vi "SetDataFolder.vi"(0 "User Data Folder":path, 2 "JustKillAllSavedReferences(False)":bool, 5 "error in (no error)":errorcluster, 6 "WebView2Control ID":i32, 8 "Webview container":refnum<k24>) -> (14 "Environment":refnum<k24>, 15 "UserDataFolder":string="C:\\ProgramData\\LcWebVIEW", 16 "Error Message":string, 19 "error out":errorcluster)   [LabVIEW 2020, in "DP_WebView.lvclass"]
uses:
  DP_WebView.lvclass
  C:/Projects/DependencyViewer/DependencyViewer/DP_WebView_class/data/Microsoft.Web.WebView2.Core.dll
  data/Microsoft.Web.WebView2.Core.dll
  C:/Projects/DependencyViewer/DependencyViewer/DP_WebView_class/data/Microsoft.Web.WebView2.WinForms.dll
  data/Microsoft.Web.WebView2.WinForms.dll
  <vilib>/Utility/sysdir.llb/System Directory Type.ctl
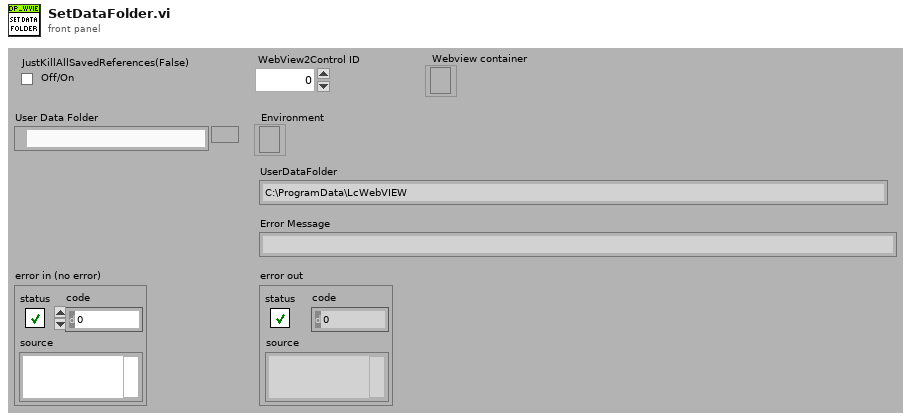
[diagram p1: front panel]
types:
  T1 = typedef "System Directory Type.ctl" = i32
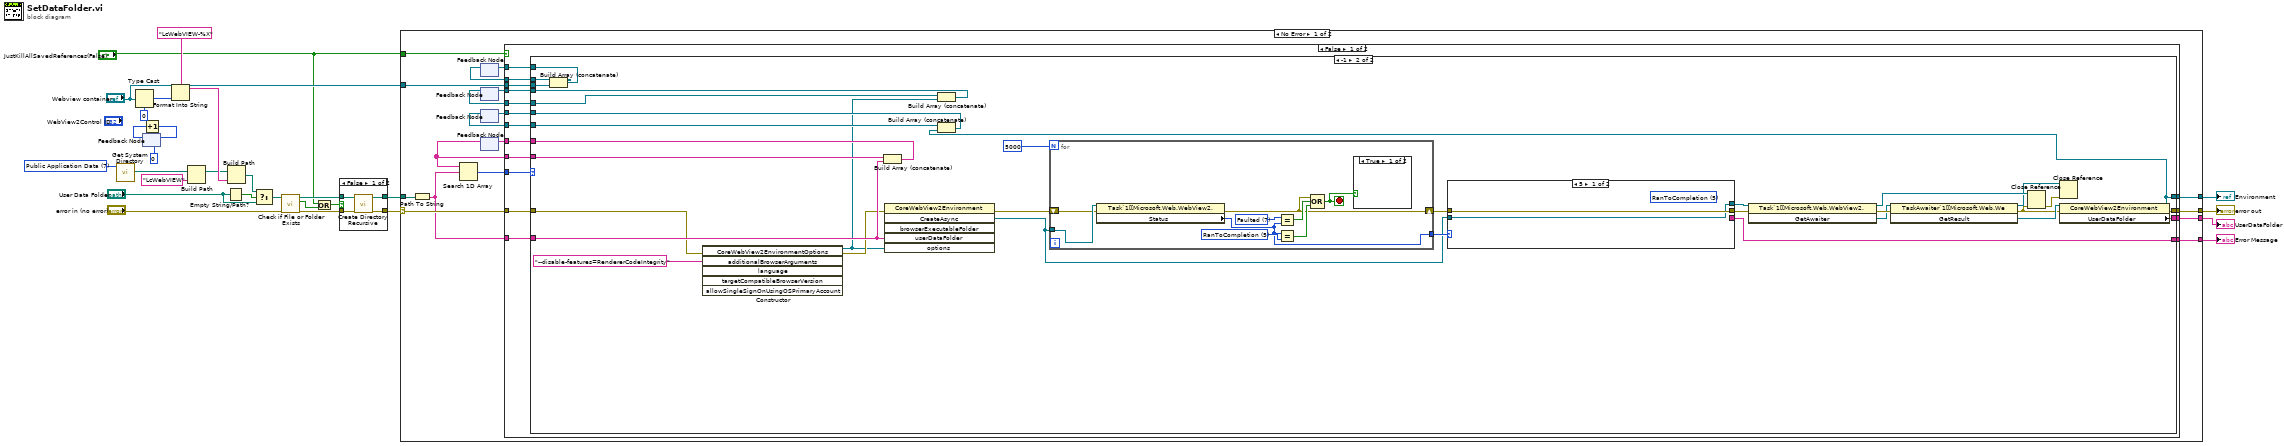
[diagram p0: block diagram]
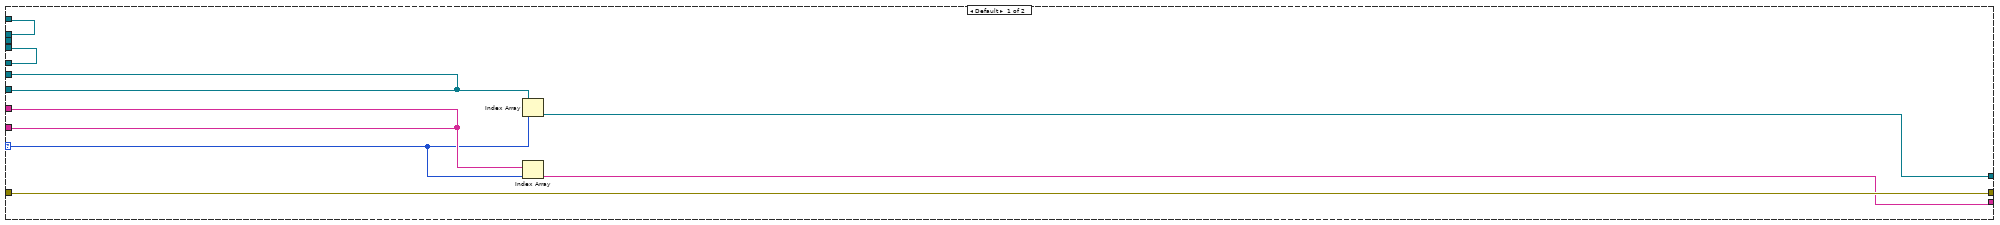
[diagram p3: hidden frame]
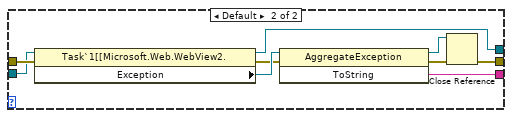
[diagram p4: hidden frame]
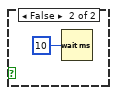
[diagram p5: hidden frame]
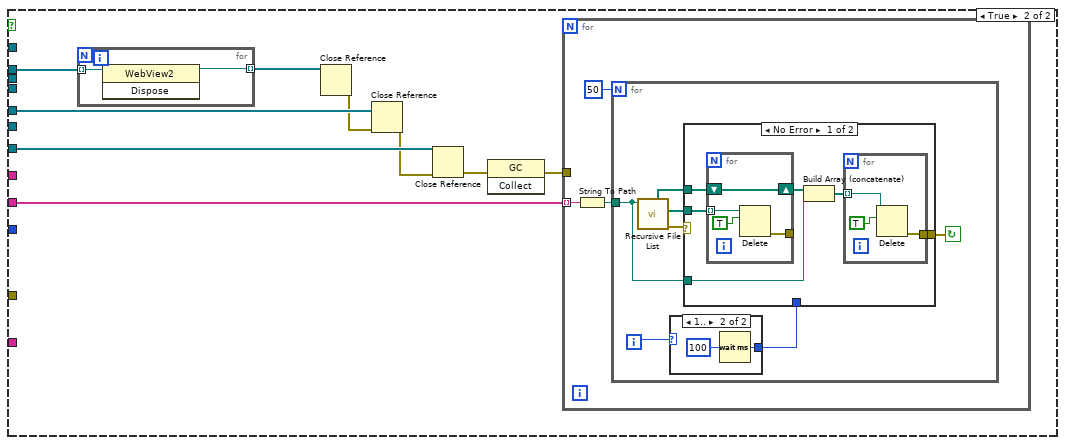
[diagram p6: hidden frame]
diagram:
  w25 = T1 7 items=["User Home"=0, "User Desktop"=1, "User Documents"=2, "User Application Data"=3, "User Preferences"=4, "User Temporary"=5, "Public Documents"=6, "Public Application Data"=7, "Public Preferences"=8, "Public Cache"=13, "System Core Libraries"=9, "System Installed Libraries"=10, "Application Files"=11, "Boot Volume Root"=12] ("system directory type")
  n1 = call <vilib>:"Get System Directory.vi"("system directory type"=w25) -> ("system directory"=w11:path)  [unwired: 10 in]
  n2 = Type Cast(type=u32 0 ("WebView2Control ID"), x="Webview container") -> (*(type *) &x=w4:u32)
  n3 = feedback #1(u32 0 ("WebView2Control ID")) -> (w7:u32)
  n4 = Increment(x=w7) -> (x+1=w6:u32)
  n5 = feedback-in #1(w6) -> ()
  n6 = Format Into String(format string="LcWebVIEW-%X", w4) -> (resulting string=w12:string)  [unwired: 2 in, 1 out]
  n7 = Build Path(base path=w11, name or relative path="LcWebVIEW") -> (appended path=w10:path)
  n8 = Empty String/Path?(string/path="User Data Folder") -> (empty?=w17:bool)
  n9 = Build Path(base path=w10, name or relative path=w12) -> (appended path=w15:path)
  n10 = Select(t=w15, s=w17, f="User Data Folder") -> (s? t:f=w14:path)
  n11 = call <vilib>:"Check if File or Folder Exists.vi"("error in (no error)"="error in (no error)", "path"=w14) -> ("error out"=w28:errorcluster, "file or folder exists?"=w26:bool, "dup path"=w27:path)  [unwired: 7 in]
  n12 = Or(x="JustKillAllSavedReferences(False)", y=w26) -> (x .or. y?=w2:bool)
  n13 = case shown="False" w2 {
    tunnel: w27 -> [w32 w33]
    tunnel: w28 -> [w31 w34]
    tunnel: [w30 w34] -> w23
    tunnel: [w29 w33] -> w22
    frame False {
      n14 = call <vilib>:"Create Directory Recursive.vi"("error in (no error)"=w31, "directory"=w32) -> ("error out"=w30:errorcluster, "directory copy"=w29:path)  [unwired: 3 in, 1 out]
    }
    frame True {
    }
  }
  n15 = case shown="No Error" w23 {
    selector: w23 -> [w52 w166]
    tunnel: w22 -> [w51 _]
    tunnel: [w49 w166] -> w21
    tunnel: [w50 _] -> w20
    tunnel: [w47 _] -> w19
    tunnel: [w48 _] -> w18
    tunnel: "JustKillAllSavedReferences(False)" -> [w38 _]
    tunnel: "Webview container" -> [w35 _]
    frame No Error {
      n16 = Path To String(path=w51) -> (string=w46:string)
      n17 = feedback #2() -> (w36:refnum<k24>[])  [unwired: 1 in]
      n18 = feedback #3() -> (w39:refnum<k24>[])  [unwired: 1 in]
      n19 = feedback #4() -> (w42:refnum<k24>[])  [unwired: 1 in]
      n20 = feedback #5() -> (w44:string[])  [unwired: 1 in]
      n21 = Search 1D Array(1D array=w44, element=w46) -> (index of element=w45:i32)  [unwired: 1 in]
      n22 = case shown="False" w38 {
        tunnel: w52 -> [w68 _]
        tunnel: [w67 _] -> w50
        tunnel: [w66 _] -> w49
        tunnel: [w65 _] -> w48
        tunnel: [w64 _] -> w47
        tunnel: w46 -> [w63 _]
        tunnel: w45 -> [w62 _]
        tunnel: w44 -> [w61 w133]
        tunnel: [w60 _] -> w43
        tunnel: w42 -> [w59 w138]
        tunnel: [w58 _] -> w41
        tunnel: [w57 _] -> w40
        tunnel: w39 -> [w56 w137]
        tunnel: [w54 _] -> w37
        tunnel: w36 -> [w55 w136]
        tunnel: w35 -> [w53 _]
        frame False {
          n23 = case shown="-1" w62 {
            selector: w62 -> [w72 _]
            tunnel: w68 -> [w74 w77]
            tunnel: [w71 w108] -> w67
            tunnel: [w74 w101] -> w66
            tunnel: [w75 w86] -> w65
            tunnel: [_ w99] -> w64
            tunnel: w63 -> [_ w92]
            tunnel: w61 -> [w73 w93]
            tunnel: [w73 w91] -> w60
            tunnel: w59 -> [w76 w90]
            tunnel: [w76 w89] -> w58
            tunnel: w56 -> [w70 w85]
            tunnel: [w70 w81] -> w57
            tunnel: w55 -> [w69 w84]
            tunnel: [w69 w82] -> w54
            tunnel: w53 -> [_ w83]
            frame Default {
              n24 = Index Array(array=w76, index=w72) -> (element=w75:refnum<k24>)
              n25 = Index Array(array=w73, index=w72) -> (element=w71:string)
            }
            frame -1 {
              n26 = Build Array (concatenate)(w84, w83) -> (w82:refnum<k24>[])
              n27 = constructor class="CoreWebView2EnvironmentOptions"(error in=w77, "additionalBrowserArguments"="--disable-features=RendererCodeIntegrity" ("AdditionalBrowserArguments")) -> (reference out=w79:refnum<k24>, error out=w87:errorcluster)  [unwired: 5 in, 5 out]
              n28 = Build Array (concatenate)(w93, w92) -> (w91:string[])
              n29 = invoke class="CoreWebView2Environment" method="CreateAsync"(error in=w87, "userDataFolder"=w92, "options"=w79) -> (error out=w78:errorcluster, "CreateAsync"=w80:refnum<k24>)  [unwired: 3 in, 4 out]
              n30 = Build Array (concatenate)(w85, w79) -> (w81:refnum<k24>[])
              n31 = for {
                N: 5000 -> [_]
                tunnel: w80 -> [w128]
                shift-right: [w122] -> w100
                shift-left: w78 -> [w127]
                tunnel: [w121] -> w96
                stop <- w120 stop-if-true
                w125 = 5 items=["Created", "WaitingForActivation", "WaitingToRun", "Running", "WaitingForChildrenToComplete", "RanToCompletion", "Canceled", "Faulted"] ("Status")
                w126 = 7 items=["Created", "WaitingForActivation", "WaitingToRun", "Running", "WaitingForChildrenToComplete", "RanToCompletion", "Canceled", "Faulted"] ("Status")
                n32 = property class="Task`1[[Microsoft.Web.WebView2."(reference=w128, error in=w127) -> (error out=w122:errorcluster, "Status"=w121:i32)  [unwired: 1 out]
                n33 = Equal?(x=w126, y=w121) -> (x = y?=w124:bool)
                n34 = Equal?(x=w121, y=w125) -> (x = y?=w123:bool)
                n35 = Compound Arithmetic op=OR(w122, w124, w123) -> (w120:bool)
                n36 = case shown="True" w120 {
                  frame True {
                  }
                  frame False {
                    n37 = Wait (ms)(milliseconds to wait=u32 10) -> ()  [unwired: 1 out]
                  }
                }
              }
              n38 = case shown="5" w96 {
                tunnel: w100 -> [w110 w119]
                tunnel: [_ w118] -> w99
                tunnel: [w110 w111] -> w98
                tunnel: w80 -> [w109 w116]
                tunnel: [w109 w115] -> w97
                frame 5 {
                  (unwired) 5 items=["Created", "WaitingForActivation", "WaitingToRun", "Running", "WaitingForChildrenToComplete", "RanToCompletion", "Canceled", "Faulted"] ("Status")
                }
                frame Default {
                  n39 = property class="Task`1[[Microsoft.Web.WebView2."(reference=w116, error in=w119) -> (reference out=w115:refnum<k24>, error out=w112:errorcluster, "Exception"=w117:refnum<k24>)
                  n40 = invoke class="AggregateException" method="ToString"(reference=w117, error in=w112) -> (reference out=w114:refnum<k24>, error out=w113:errorcluster, "ToString"=w118:string)  [unwired: 1 in]
                  n41 = Close Reference(reference=w114, error in (no error)=w113) -> (error out=w111:errorcluster)
                }
              }
              n42 = invoke class="Task`1[[Microsoft.Web.WebView2." method="GetAwaiter"(reference=w97, error in=w98) -> (reference out=w103:refnum<k24>, error out=w106:errorcluster, "GetAwaiter"=w104:refnum<k24>)  [unwired: 1 in]
              n43 = invoke class="TaskAwaiter`1[[Microsoft.Web.We" method="GetResult"(reference=w104, error in=w106) -> (reference out=w94:refnum<k24>, error out=w102:errorcluster, "GetResult"=w105:refnum<k24>)  [unwired: 1 in]
              n44 = Close Reference(reference=w103, error in (no error)=w102) -> (error out=w95:errorcluster)
              n45 = Close Reference(reference=w94, error in (no error)=w95) -> ()  [unwired: 1 out]
              n46 = property class="CoreWebView2Environment"(reference=w105, error in=w102) -> (reference out=w86:refnum<k24>, error out=w101:errorcluster, "UserDataFolder"=w108:string)
              n47 = Build Array (concatenate)(w90, w86) -> (w89:refnum<k24>[])
            }
          }
        }
        frame True {
          n48 = for {
            tunnel: w136 -> [w165] mode=indexing
            tunnel: [w164] -> w135 mode=indexing
            n49 = invoke class="WebView2" method="Dispose"(reference=w165) -> (reference out=w164:refnum<k24>)  [unwired: 2 in, 2 out]
          }
          n50 = Close Reference(reference=w135) -> (error out=w132:errorcluster)  [unwired: 1 in]
          n51 = Close Reference(reference=w137, error in (no error)=w132) -> (error out=w131:errorcluster)
          n52 = Close Reference(reference=w138, error in (no error)=w131) -> (error out=w130:errorcluster)
          n53 = invoke class="GC" method="Collect"(error in=w130) -> (error out=w134:errorcluster)  [unwired: 2 in, 2 out]
          n54 = for {
            tunnel: w134 -> [_]
            tunnel: w133 -> [w141] mode=indexing
            n55 = String To Path(string=w141) -> (path=w140:path)
            n56 = for {
              N: 50 -> [_]
              tunnel: w140 -> [w146]
              i -> [w143]
              stop <- w145 continue-if-true
              n57 = call <vilib>:"Recursive File List.vi"("Folder Path"=w146) -> ("error out"=w144:errorcluster, "All Files in Dir"=w148:path[], "All Folders"=w147:path[])  [unwired: 6 in, 2 out]
              n58 = case shown="1.." w143 {
                tunnel: [_ w149] -> w142
                frame 0, Default {
                }
                frame 1.. {
                  n59 = Wait (ms)(milliseconds to wait=u32 100) -> (millisecond timer value=w149:u32)
                }
              }
              n60 = case shown="No Error" w144 {
                tunnel: w148 -> [w156 _]
                tunnel: w147 -> [w154 _]
                tunnel: w146 -> [w152 _]
                tunnel: [w151 _] -> w145
                tunnel: w142 -> [_ _]
                frame No Error {
                  n61 = for {
                    tunnel: w156 -> [w162] mode=indexing
                    tunnel: [w160] -> _
                    shift-right: [w161] -> w155
                    shift-left: w154 -> [w161]
                    n62 = Delete(path (use dialog)=w162, entire hierarchy (F)=TRUE) -> (error out=w160:errorcluster)  [unwired: 3 in, 2 out]
                  }
                  n63 = Build Array (concatenate)(w155, w152) -> (w153:path[])
                  n64 = for {
                    tunnel: w153 -> [w158] mode=indexing
                    tunnel: [w157] -> w151
                    n65 = Delete(path (use dialog)=w158, entire hierarchy (F)=TRUE) -> (error out=w157:errorcluster)  [unwired: 3 in, 2 out]
                  }
                }
                frame Error {
                  # "All files gone :-)"
                }
              }
            }
          }
        }
      }
      n66 = feedback-in #2(w37) -> ()
      n67 = feedback-in #3(w40) -> ()
      n68 = feedback-in #4(w41) -> ()
      n69 = feedback-in #5(w43) -> ()
    }
    frame Error {
    }
  }
  "error out" <- w21
  "UserDataFolder" <- w20
  "Error Message" <- w19
  "Environment" <- w18
